vi "CopieExcelFile.vi"(3 "Entrée d'erreur":errorcluster, 5 "NomProjet":string) -> (0 "sortie d'erreur":errorcluster, 2 "NomProjetOut":string)   [LabVIEW 2017]
uses:
  DefDeType/WhichPath.ctl
panel:
  out "fichier destination":path
  out "fichier source":path
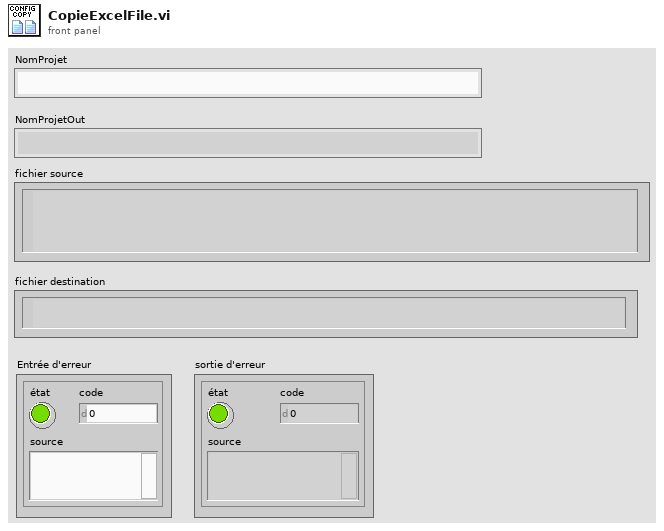
[diagram p1: front panel]
types:
  T1 = typedef "WhichPath.ctl" = enum16{"DossierProjet", "Config", "Meas", "MeasPCI", "MeasCRIO1", "MeasCRIO2", "MeasQualisys", "MeasHBM", "MeasTDMS", "Fig", "Res"}
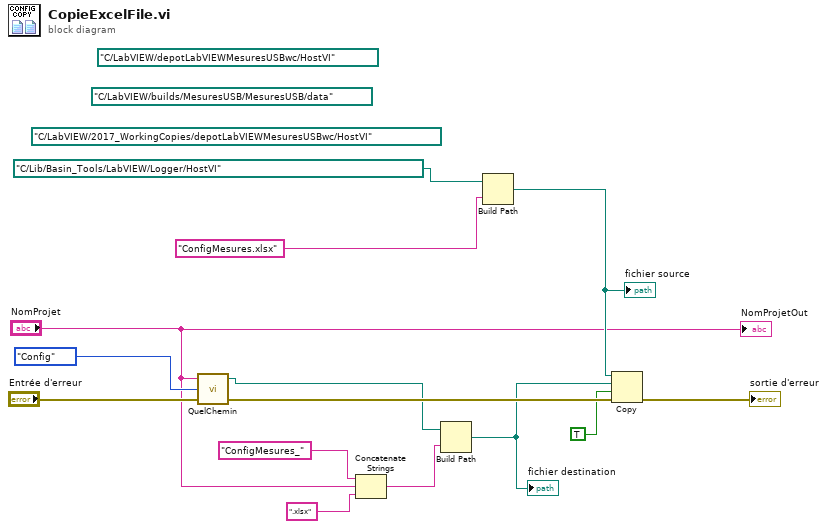
[diagram p0: block diagram]
diagram:
  (unwired) path "C:/LabVIEW/2017_WorkingCopies/depotLabVIEWMesuresUSBwc/HostVI" ("appended path 2")
  (unwired) path "C:/LabVIEW/depotLabVIEWMesuresUSBwc/HostVI" ("appended path 2")
  (unwired) path "C:/LabVIEW/builds/MesuresUSB/MesuresUSB/data" ("appended path 2")
  n1 = call "QuelChemin.vi"("Entrée d'erreur"="Entrée d'erreur", "WhichPath?"=WhichPath."Config", "NomProjet"="NomProjet") -> ("Sortie d'erreur"=w13:errorcluster, "SurDisqueLocal"=w4:path)  [unwired: 1 out]
  n2 = Concatenate Strings("ConfigMesures_" ("nom ou chemin relatif"), "NomProjet", ".xlsx" ("nom ou chemin relatif")) -> (w3:string)
  n3 = Build Path(base path=w4, name or relative path=w3) -> (appended path=w2:path)
  "fichier destination" <- w2
  n4 = Build Path(base path=path "C:/Lib/Basin_Tools/LabVIEW/Logger/HostVI" ("appended path 2"), name or relative path="ConfigMesures.xlsx" ("nom ou chemin relatif")) -> (appended path=w14:path)
  "fichier source" <- w14
  n5 = Copy(8:w13, 9:TRUE ("écraser (F)"), 10:w2, 11:w14) -> (0:→"sortie d'erreur":errorcluster)  [unwired: 1 in, 2 out]
  "NomProjetOut" <- "NomProjet"
